vi "Get_Quaternion.vi"(5 "Device Number":T1, 7 "Update":bool) -> (2 "Quaternion":T2)   [LabVIEW 2019]
doc: "This navX VI returns the quaternion of the navX."
uses:
  _TypeDefs/FRIC_navX_DeviceNumbersTypeDef.ctl
  _TypeDefs/Z900_navX_DeviceRegisters.ctl
  _Util/Z900_navX_Util_LittleEndian_to_BigEndian.vi
  _Internal/FRIC_navX_Get_Registry.vi
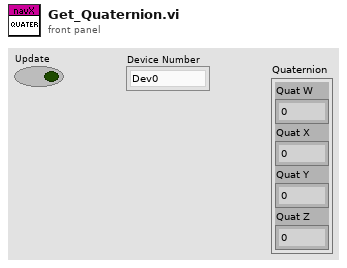
[diagram p1: front panel]
types:
  T1 = typedef "FRIC_navX_DeviceNumbersTypeDef.ctl" = enum16{"Dev0", "Dev1", "Dev2", "Dev3"}
  T2 = cluster{"Quat W":dbl, "Quat X":dbl, "Quat Y":dbl, "Quat Z":dbl}
  T3 = typedef "Z900_navX_DeviceRegisters.ctl" = u8
  T4 = typedef "Z900_navX_ProtocolTypeDef.ctl" = enum16{"SERIAL", "I2C", "SPI"}
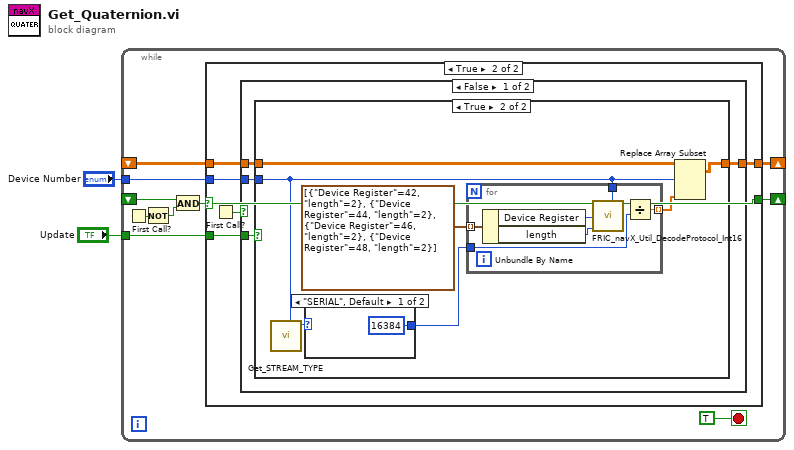
[diagram p0: block diagram]
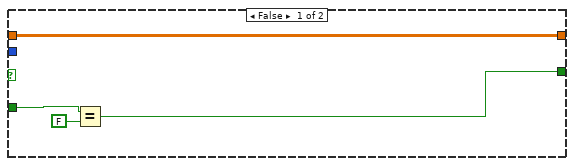
[diagram p2: hidden frame]
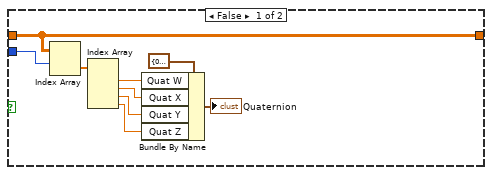
[diagram p3: hidden frame]
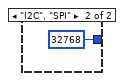
[diagram p4: hidden frame]
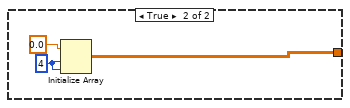
[diagram p5: hidden frame]
diagram:
  n1 = while {
    shift-right: [w12] -> _
    shift-left: _ -> [w11]
    tunnel: "Update" -> [w9]
    tunnel: "Device Number" -> [w8]
    shift-right: [w3] -> _
    shift-left: _ -> [w5]
    stop <- TRUE stop-if-true
    n2 = First Call?() -> (First Call?: T/F=w6:bool)
    n3 = Not(x=w6) -> (.not. x?=w7:bool)
    n4 = And(x=w5, y=w7) -> (x .and. y?=w4:bool)
    n5 = case shown="True" w4 {
      selector: w4 -> [_ w17]
      tunnel: [w13 w22] -> w12
      tunnel: w11 -> [w13 w21]
      tunnel: w9 -> [w15 w20]
      tunnel: w8 -> [_ w19]
      tunnel: [w14 w17] -> w3
      frame False {
        n6 = Equal?(x=w15, y=FALSE) -> (x = y?=w14:bool)
      }
      frame True {
        n7 = First Call?() -> (First Call?: T/F=w18:bool)
        n8 = case shown="False" w18 {
          tunnel: [w26 w54] -> w22
          tunnel: w21 -> [w25 _]
          tunnel: w20 -> [w23 _]
          tunnel: w19 -> [w24 _]
          frame False {
            n9 = case shown="True" w23 {
              tunnel: [w34 w41] -> w26
              tunnel: w25 -> [w34 w42]
              tunnel: w24 -> [w35 w36]
              frame False {
                n10 = Index Array(array=w34, index (row)=w35) -> (element=w32:dbl[])  [unwired: 1 in]
                n11 = Index Array(array=w32) -> (element #1=w31:dbl, element #2=w30:dbl, element #3=w29:dbl, element #4=w28:dbl)  [unwired: 4 in]
                n12 = Bundle By Name(cluster=T2 {"Quat W"=0.0, "Quat X"=0.0, "Quat Y"=0.0, "Quat Z"=0.0}, "Quat W"=w31, "Quat X"=w30, "Quat Y"=w29, "Quat Z"=w28) -> (→"Quaternion":T2)
              }
              frame True {
                n13 = call "Get_STREAM_TYPE.vi"("Device Number"=w36) -> ("Protocol (out)"=w37:T4)  [unwired: 10 in]
                n14 = case shown="\"SERIAL\", Default" w37 {
                  tunnel: [u16 16384 ("y") u16 32768 ("y")] -> w39
                  frame "SERIAL", Default {
                  }
                  frame "I2C", "SPI" {
                  }
                }
                n15 = for {
                  tunnel: cluster{"Device Register":T3, "length":i32}[] [{"Device Register"=42, "length"=2}, {"Device Register"=44, "length"=2}, {"Device Register"=46, "length"=2}, {"Device Register"=48, "length"=2}] ("Array") -> [w49] mode=indexing
                  tunnel: w36 -> [w48]
                  tunnel: w39 -> [w46]
                  tunnel: [w45] -> w38 mode=indexing
                  n16 = Unbundle By Name(w49) -> ("Device Register"=w51:T3, "length"=w50:i32)
                  n17 = call "FRIC_navX_Util_DecodeProtocol_Int16.vi"("Device Number"=w48, "length"=w50, "Device Register"=w51) -> ("Value"=w47:i16)  [unwired: 8 in]
                  n18 = Divide(x=w47, y=w46) -> (x/y=w45:dbl)
                }
                n19 = Replace Array Subset(array=w42, new element=w38, index (row)=w36) -> (w41:dbl[][])  [unwired: 1 in]
              }
            }
          }
          frame True {
            w53 = 4 ("dimension size")
            n20 = Initialize Array(0.0, w53, w53) -> (w54:dbl[][])
          }
        }
      }
    }
  }
